vi "Configure Acquisition.vi"(0 "device session in":refnum<class "Device Session.lvclass">, 1 "pretrigger samples":u64, 2 "number of records is finite (T)":bool=TRUE, 5 "number of records":u64=1, 7 "number of samples":u64=1000, 9 "channels to store":u32[](array[numeric]), 11 "error in":errorcluster, 12 "additional configuration":T1={"record padding (samples)"=0, "require finite records to fit in memory"=TRUE, "timestamps per record"=1, "status fifo depth (records)"=10000}) -> (4 "device session out":refnum<class "Device Session.lvclass">, 6 "actual channels stored":bool[](array[boolean]), 15 "error out":errorcluster)   [LabVIEW 2021, in "Device Session.lvclass"]
doc: "Configures the acquisition. You can specify which channels to acquire from, how many records to acquire, and how many samples to acquire. You must run this VI before running the <B>Initiate</B> VI.\n\n<B>Input Parameters</B>\n\n<B>device session in</B> is a reference to the Device Session object, which contains a session to each instrument design library used in this sample project. This parameter is obtained from the 'Open Session' VI.\n\n<B>number of records is finite (T)</B> specifies whether to acquire a finite number of records, or to acquire records continuously.\n\n<B>pretrigger samples</B> specifies, for every record, the minimum number of samples that must be stored from the time period immediately before the Reference Trigger occurred.\n\n<B>number of records</B> specifies the number of records to acquire. The default value is 1.\n\n<B>number of samples</B> specifies the number of samples to acquire. The default value is 1000.\n\n<B>channels to store</B> specifies the channels to store in memory. By default, only the channels configured using the 'Configure Channel' VI are stored.\n\n<B>additional configuration</B> specifies additional advanced configurations.\n\n<B>additional configuration.record padding (samples)</B> specifies additional padding to allocate for a record. This parameter can be useful in combination with adjusting the Reference Trigger position. The default value is 0.\n\n<B>additional configuration.require finite records to fit in memory</B> specifies that the requested number of records and samples must fit into memory for finite acquisitions. This parameter ensures that requested data cannot be overwritten for finite acquisitions. The default is TRUE.\n\n<B>additional configuration.timestamps per record</B> specifies the number of timestamp values the FPGA captures for each record. This value must match the number of timestamps per record provided to the Write VI of the Multirecord Acquisition FPGA library. The default value is 0.\n\n<B>additional configuration.status fifo depth (records)</B> Sets the depth of the record status DMA FIFO. The Status FIFO reports information about the current state of the acquisition to the host.\nEnsure that the Status FIFO is deep enough for the rate at which the host consumes this FIFO. If the Status FIFO is full, memory writes are delayed. Eventually, this can cause the Write FIFO to fill up and overflow. The host consumes the entire Status FIFO each time you fetch a record or query acquisition status. The value is specified in units of records. The default value is 10,000 records.\n\n<B>error in</B> describes error conditions that occur before this node runs. This input provides standard 'error in' functionality.\n\n<B>Output Parameters</B>\n\n<B>device session out</B> passes a reference to the session to the next VI.\n\n<B>actual channels stored</B> returns the number of channels stored as a power of two.\n\n<B>error out</B> contains error information. This output provides standard 'error out' functionality."
uses:
  Device Session.lvclass
  <instrlib>/_niInstr/Multirecord Acquisition/Interface/v1/Host/Public/Additional Acquisition Configuration.ctl
  Device Session.lvclass/Device Session.ctl
  <vilib>/Utility/error.llb/Error Cluster From Error Code.vi
  <vilib>/rvi/errors/niLvFpgaAdjustHostInterfaceError.vi
  <vilib>/rvi/interface/nirviReadWriteControl/nirviReadWriteControl.xnode
  FPGA Refnum.ctl
  <instrlib>/_niInstr/Multirecord Acquisition/Interface/v1/Host/niInstr Multirecord Acquisition v1 Host.lvclass
  <vilib>/rvi/interface/Simulation/niFpgaSimulationCallBeginRW.vi
  NiFpgaLv.dll
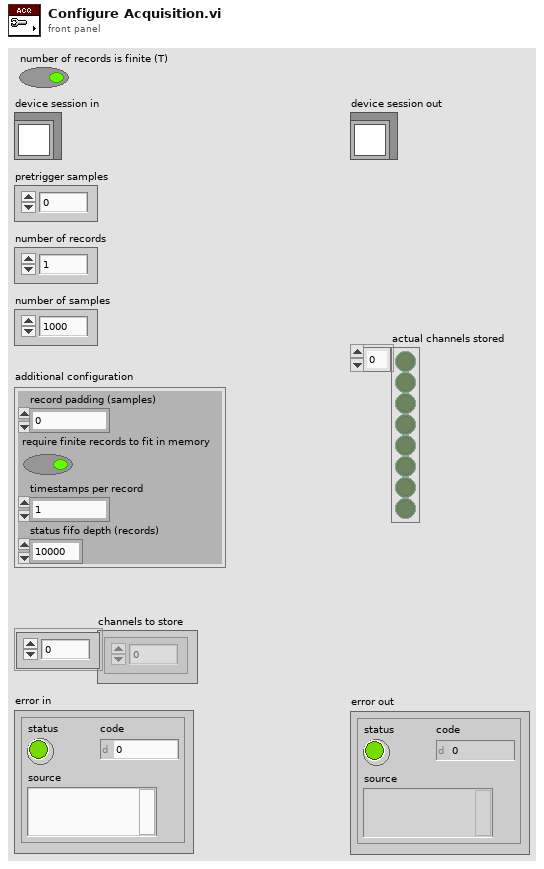
[diagram p1: front panel]
types:
  T1 = typedef "niInstr Multirecord Acquisition v1 Host.lvclass/Additional Acquisition Configuration.ctl" = cluster{"record padding (samples)":u64, "require finite records to fit in memory":bool, "timestamps per record":u32, "status fifo depth (records)":u32}
  T2 = typedef "Device Session.lvclass/Device Session Object.ctl" = cluster{"fpga reference":T3, "reg bus":refnum<class "niInstr FIFO Register Bus v1 Host.lvclass">, "subsystem map":refnum<class "niInstr Subsystem Map v1 Host.lvclass">, "cal data":refnum<class "niHSAI Cal Data v1 Host.lvclass">, "config":refnum<class "niHSAI Group A Config v1 Host.lvclass">, "acquisition 0":refnum<class "niInstr Multirecord Acquisition v1 Host.lvclass">, "acquisition 1":refnum<class "niInstr Multirecord Acquisition v1 Host.lvclass">, "number of selected acq channels":u8, "selected acq channels":bool[], "number of channels":u32, "configured channels":bool[], "acq configuration":cluster{"number of samples":u64, "number of records":u64, "pretrigger samples":u64}, "actual channel configuration":T4[], "sample clock rate (Hz)":dbl, "scaling coefficients":T8[]}
  T3 = typedef "Device Session.lvclass/FPGA Refnum.ctl" = refnum<k20>
  T4 = typedef "niHSAI Types v1 Host.lvlib/Channel Configuration.ctl" = cluster{"channel":u32, "coupling":T5, "impedance":T6, "bandwidth":T7, "vertical range":dbl, "vertical offset":dbl}
  T5 = typedef "niHSAI Types v1 Host.lvlib/Coupling.ctl" = enum8{"Default", "DC", "AC"}
  T6 = typedef "niHSAI Types v1 Host.lvlib/Impedance.ctl" = enum8{"Default", "1 mega ohm", "50 ohm"}
  T7 = typedef "niHSAI Types v1 Host.lvlib/Bandwidth.ctl" = enum8{"Default", "Full Bandwidth", "Anti-alias Filter", "150 MHz"}
  T8 = typedef "niInstr Multirecord Acquisition v1 Host.lvclass/Scaling Coefficient.ctl" = cluster{"gain":dbl, "offset":dbl}
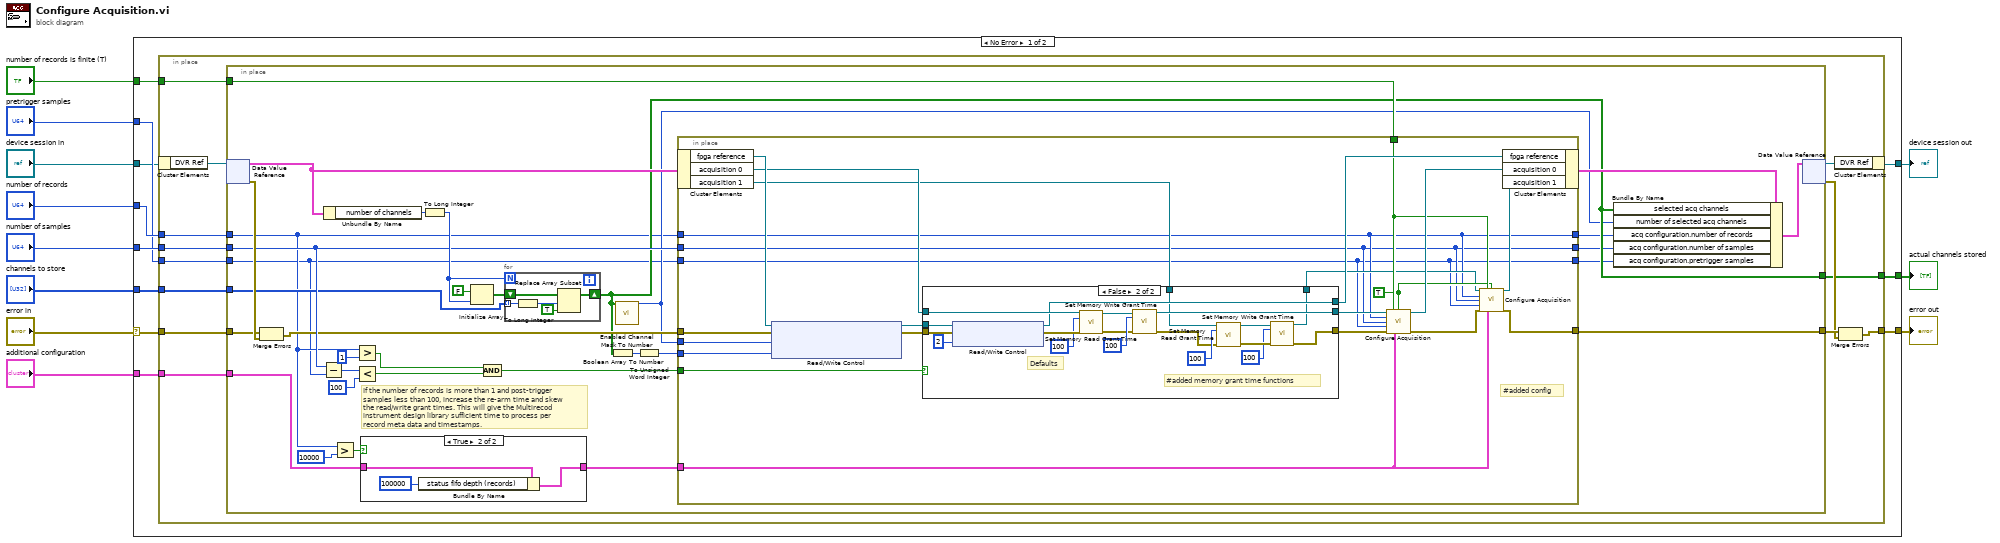
[diagram p0: block diagram]
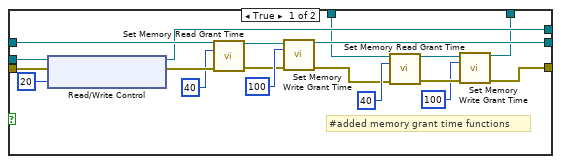
[diagram p2: hidden frame]
diagram:
  n1 = case shown="No Error" "error in" {
    selector: "error in" -> [w22 w140]
    tunnel: [w14 w140] -> w10
    tunnel: "device session in" -> [w12 w139]
    tunnel: [w13 w139] -> w8
    tunnel: "number of records" -> [w21 _]
    tunnel: "number of samples" -> [w20 _]
    tunnel: "channels to store" -> [w19 _]
    tunnel: [w18 _] -> w4
    tunnel: "pretrigger samples" -> [w17 _]
    tunnel: "additional configuration" -> [w16 _]
    tunnel: "number of records is finite (T)" -> [w15 _]
    frame No Error {
      n2 = in-place {
        in-place-border: w22 -> [w35]
        in-place-border: w21 -> [w34]
        in-place-border: w20 -> [w33]
        in-place-border: w19 -> [w30]
        in-place-border: [w29] -> w18
        in-place-border: w17 -> [w28]
        in-place-border: w16 -> [w27]
        in-place-border: w15 -> [w26]
        in-place-border: [w25] -> w14
        n3 = in-place-cluster #1(w12) -> ("DVR Ref"=w24:refnum<data-value>)
        n4 = in-place {
          in-place-border: w35 -> [w63]
          in-place-border: [w66] -> w32
          in-place-border: w34 -> [w37]
          in-place-border: w33 -> [w49]
          in-place-border: w30 -> [w38]
          in-place-border: [w43] -> w29
          in-place-border: w28 -> [w36]
          in-place-border: w27 -> [w47]
          in-place-border: w26 -> [w60]
          # "If the number of records is more than 1 and post-trigger samples less than 100, increase the re-arm time and skew the read/write grant times. This will give the Multirecod instrument design library sufficient time to process per record meta data and timestamps."
          n5 = in-place-dvr #2(w24) -> (w45:T2, w67:errorcluster)
          n6 = Merge Errors(w63, w67) -> (w48:errorcluster)
          n7 = Subtract(x=w49, y=w36) -> (x-y=w57:u64)
          n8 = Unbundle By Name(w45) -> ("number of channels"=w59:u32)
          n9 = Greater?(x=w37, y=u64 10000) -> (0:w50:bool)
          n10 = Greater?(x=w37, y=u64 1) -> (0:w54:bool)
          n11 = Less?(x=w57, y=u64 100) -> (x < y?=w53:bool)
          n12 = case shown="True" w50 {
            tunnel: w47 -> [w130 w133]
            tunnel: [w130 w131] -> w46
            frame False {
            }
            frame True {
              n13 = Bundle By Name(cluster=w133, "status fifo depth (records)"=u32 100000) -> (w131:T1)
            }
          }
          n14 = To Long Integer(number=w59) -> (32bit integer=w58:i32)
          n15 = Initialize Array(FALSE, w58) -> (w61:bool[])
          n16 = And(x=w54, y=w53) -> (x .and. y?=w52:bool)
          n17 = for {
            N: w58 -> [_]
            tunnel: w38 -> [w135] mode=indexing
            shift-right: [w137] -> w43
            shift-left: w61 -> [w136]
            n18 = To Long Integer(number=w135) -> (32bit integer=w134:i32)
            n19 = Replace Array Subset(array=w136, new element=TRUE ("new element/subarray"), index=w134) -> (w137:bool[])
          }
          n20 = Boolean Array To Number(Boolean array=w43) -> (number=w65:u32)
          n21 = call "Enabled Channel Mask To Number.vi"("selected acquisition channels to store"=w43) -> ("number of selected channels"=w42:u8)  [unwired: 14 in]
          n22 = To Unsigned Word Integer(number=w65) -> (unsigned 16bit integer=w64:u16)
          n23 = in-place {
            in-place-border: [w73] -> w66
            in-place-border: w64 -> [w91]
            in-place-border: w60 -> [w78]
            in-place-border: w52 -> [w86]
            in-place-border: w36 -> [w70]
            in-place-border: w49 -> [w71]
            in-place-border: w48 -> [w85]
            in-place-border: w37 -> [w72]
            in-place-border: w42 -> [w84]
            in-place-border: w46 -> [w69]
            in-place-border: [w72] -> w41
            in-place-border: [w71] -> w40
            in-place-border: [w70] -> w39
            w77 = TRUE ("number of samples is finite")
            # "#added config"
            n24 = in-place-cluster #3(w45) -> ("fpga reference"=w83:T3, "acquisition 0"=w82:refnum<class "niInstr Multirecord Acquisition v1 Host.lvclass">, "acquisition 1"=w79:refnum<class "niInstr Multirecord Acquisition v1 Host.lvclass">)
            n25 = xnode "Read/Write Control"("FPGA VI Reference In"=w83, "error in"=w85, "channel.number of channels"=w84, "channel.enable mask"=w91) -> ("FPGA VI Reference Out"=w90:T3, "error out"=w89:errorcluster)
            n26 = case shown="False" w86 {
              tunnel: w82 -> [w104 w123]
              tunnel: w90 -> [w105 w124]
              tunnel: w89 -> [w103 w122]
              tunnel: [w94 w113] -> w88
              tunnel: [w102 w121] -> w87
              tunnel: [w100 w119] -> w81
              tunnel: w79 -> [w92 w112]
              tunnel: [w93 w111] -> w76
              frame True {
                # "#added memory grant time functions"
                n27 = xnode "Read/Write Control"("FPGA VI Reference In"=w105, "error in"=w103, "trigger.rearm delay"=u16 20 ("trigger.rearm time")) -> ("FPGA VI Reference Out"=w100:T3, "error out"=w110:errorcluster)
                n28 = call-dynamic "Set Memory Read Grant Time.vi"("session in"=w104, "grant time (clocks)"=u32 40, "error in"=w110) -> ("session out"=w106:refnum<class "niInstr Multirecord Acquisition v1 Host.lvclass">, "error out"=w107:errorcluster)  [unwired: 11 in]
                n29 = call-dynamic "Set Memory Write Grant Time.vi"("session in"=w106, "grant time (clocks)"=u32 100, "error in"=w107) -> ("session out"=w102:refnum<class "niInstr Multirecord Acquisition v1 Host.lvclass">, "error out"=w95:errorcluster)  [unwired: 11 in]
                n30 = call-dynamic "Set Memory Read Grant Time.vi"("session in"=w92, "grant time (clocks)"=u32 40, "error in"=w95) -> ("session out"=w99:refnum<class "niInstr Multirecord Acquisition v1 Host.lvclass">, "error out"=w98:errorcluster)  [unwired: 11 in]
                n31 = call-dynamic "Set Memory Write Grant Time.vi"("session in"=w99, "grant time (clocks)"=u32 100, "error in"=w98) -> ("session out"=w93:refnum<class "niInstr Multirecord Acquisition v1 Host.lvclass">, "error out"=w94:errorcluster)  [unwired: 11 in]
              }
              frame False {
                # "#added memory grant time functions"
                # "Defaults"
                n32 = xnode "Read/Write Control"("FPGA VI Reference In"=w124, "error in"=w122, "trigger.rearm delay"=u16 2 ("trigger.rearm time")) -> ("FPGA VI Reference Out"=w119:T3, "error out"=w129:errorcluster)
                n33 = call-dynamic "Set Memory Read Grant Time.vi"("session in"=w123, "grant time (clocks)"=u32 100, "error in"=w129) -> ("session out"=w125:refnum<class "niInstr Multirecord Acquisition v1 Host.lvclass">, "error out"=w126:errorcluster)  [unwired: 11 in]
                n34 = call-dynamic "Set Memory Write Grant Time.vi"("session in"=w125, "grant time (clocks)"=u32 100, "error in"=w126) -> ("session out"=w121:refnum<class "niInstr Multirecord Acquisition v1 Host.lvclass">, "error out"=w114:errorcluster)  [unwired: 11 in]
                n35 = call-dynamic "Set Memory Read Grant Time.vi"("session in"=w112, "grant time (clocks)"=u32 100, "error in"=w114) -> ("session out"=w118:refnum<class "niInstr Multirecord Acquisition v1 Host.lvclass">, "error out"=w117:errorcluster)  [unwired: 11 in]
                n36 = call-dynamic "Set Memory Write Grant Time.vi"("session in"=w118, "grant time (clocks)"=u32 100, "error in"=w117) -> ("session out"=w111:refnum<class "niInstr Multirecord Acquisition v1 Host.lvclass">, "error out"=w113:errorcluster)  [unwired: 11 in]
              }
            }
            n37 = call-dynamic "Configure Acquisition.vi"("session in"=w87, "number of records is finite"=w78, "number of samples is finite"=w77, "number of records"=w72, "number of samples"=w71, "pretrigger samples"=w70, "error in"=w88, "additional acquisition configuration"=w69) -> ("session out"=w80:refnum<class "niInstr Multirecord Acquisition v1 Host.lvclass">, "error out"=w74:errorcluster)  [unwired: 5 in, 1 out]
            n38 = call-dynamic "Configure Acquisition.vi"("session in"=w76, "number of records is finite"=w78, "number of samples is finite"=w77, "number of records"=w72, "number of samples"=w71, "pretrigger samples"=w70, "error in"=w74, "additional acquisition configuration"=w69) -> ("session out"=w75:refnum<class "niInstr Multirecord Acquisition v1 Host.lvclass">, "error out"=w73:errorcluster)  [unwired: 5 in, 1 out]
            n39 = in-place-cluster #3("fpga reference"=w81, "acquisition 0"=w80, "acquisition 1"=w75) -> (w44:T2)
          }
          n40 = Bundle By Name(cluster=w44, "selected acq channels"=w43, "number of selected acq channels"=w42, "acq configuration.number of records"=w41, "acq configuration.number of samples"=w40, "acq configuration.pretrigger samples"=w39) -> (w68:T2)
          n41 = in-place-dvr #2(w68) -> (w23:refnum<data-value>, w31:errorcluster)
        }
        n42 = in-place-cluster #1("DVR Ref"=w23) -> (w13:refnum<class "Device Session.lvclass">)
        n43 = Merge Errors(w32, w31) -> (w25:errorcluster)
      }
    }
    frame Error {
    }
  }
  "error out" <- w10
  "device session out" <- w8
  "actual channels stored" <- w4
